vi "MAC6000_test.vi"() -> ()   [LabVIEW 2018, in "Stage Controller.lvlib"]
uses:
  <vilib>/Instr/_visa.llb/VISA Configure Serial Port (Instr).vi
  Stage Controller.lvlib
panel:
  out "COM Port":string
  in  "Status":bool
  in  "Controller Response":string
  in  "ABORT":bool
  in  "Tab Control":enum32{"Jump", "Home", "Scan"}(tab)
  in  "Step (um)":i32=100
  in  "Move Forward Button":bool
  in  "Move Back Button":bool
  in  "Next Lane Button":bool
  in  "Previous Lane Button":bool
  in  "Move Home":bool
  in  "Set Home":bool
  in  "Scan distance (um)":i32=1000
  in  "Scan Speed\n(pulses per sec)":u32=100 min=100 max=20000
  in  "Scan":bool
  in  "Exit":bool
  out "error out":errorcluster
  # "X Direction"
  # "µm"
  # "Y Direction"
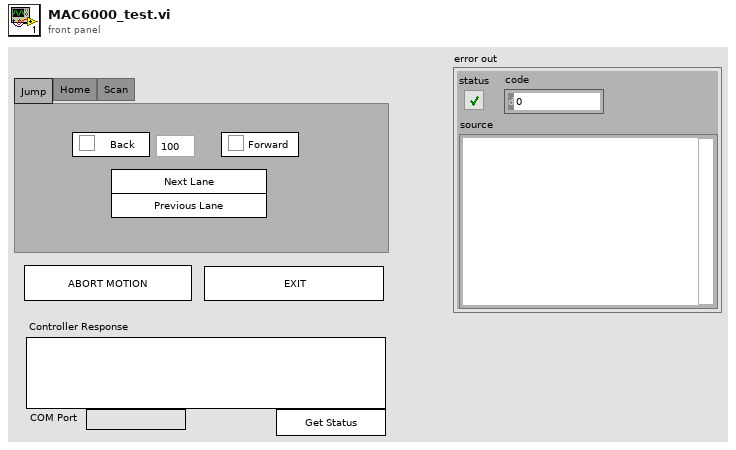
[diagram p1: front panel]
types:
  T1 = enum8{"Enabled", "Disabled", "Disabled and Grayed Out"}
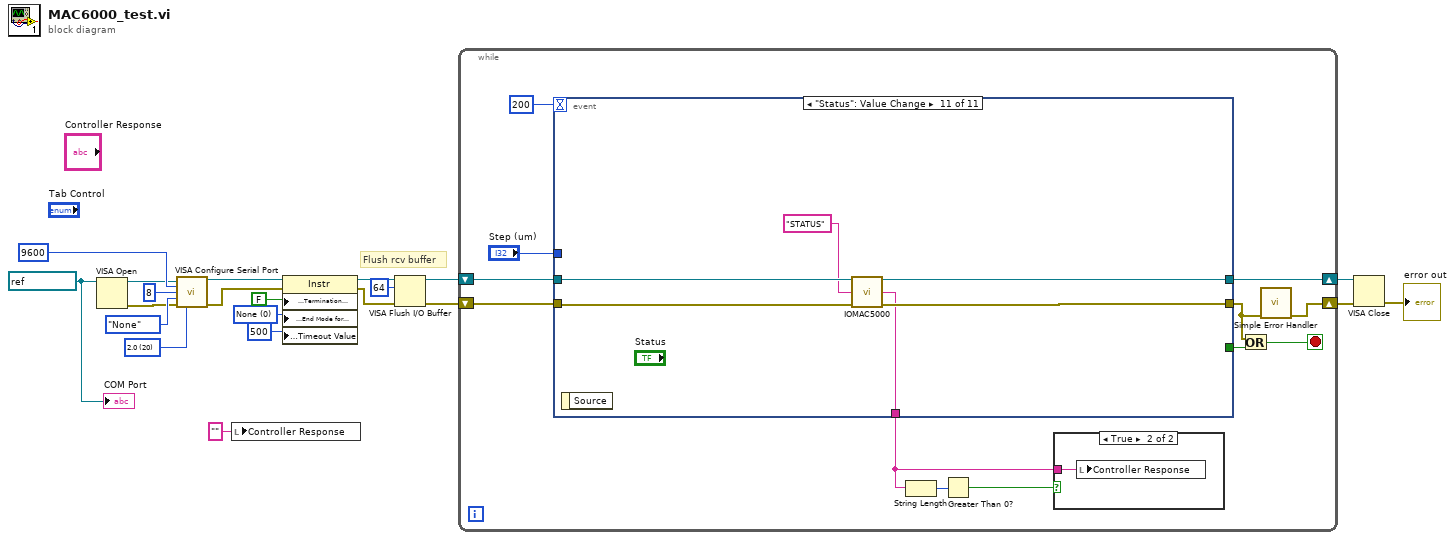
[diagram p0: block diagram]
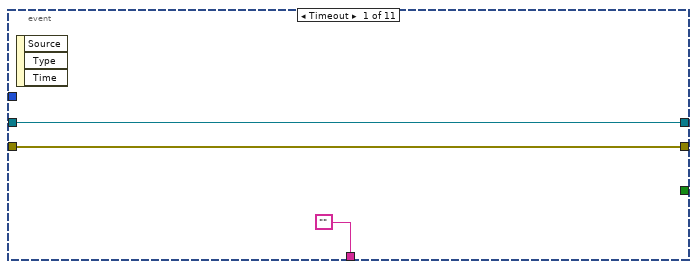
[diagram p3: hidden frame]
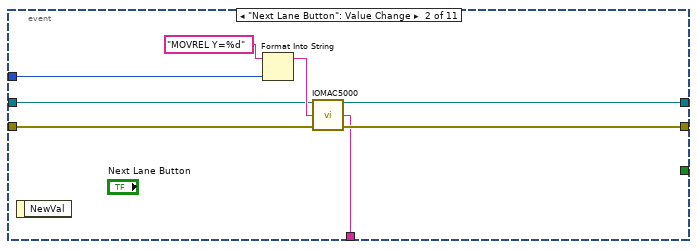
[diagram p4: hidden frame]
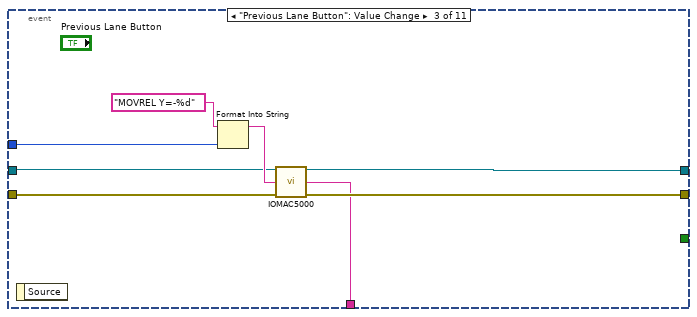
[diagram p5: hidden frame]
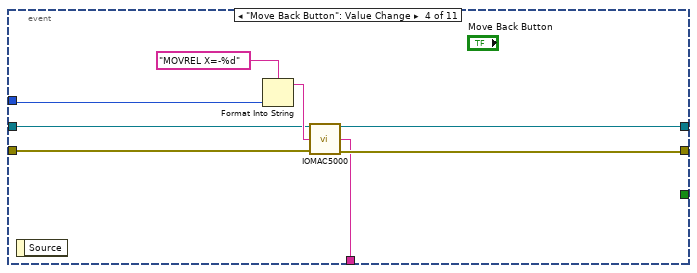
[diagram p6: hidden frame]
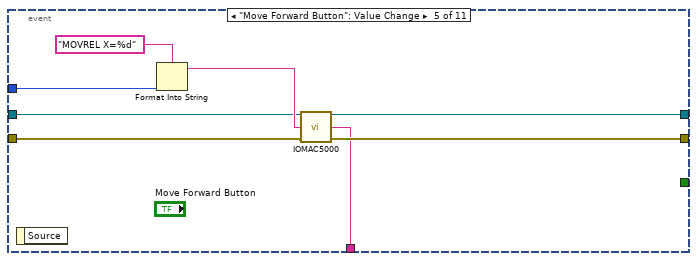
[diagram p7: hidden frame]
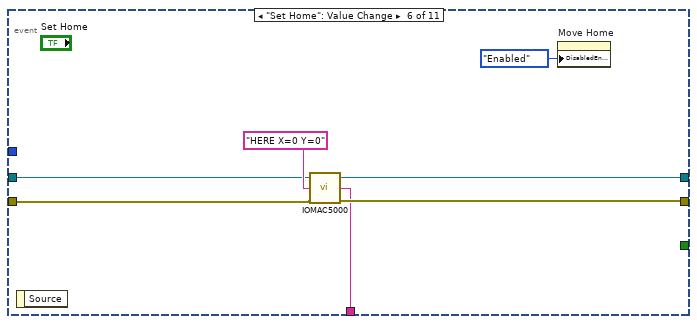
[diagram p8: hidden frame]
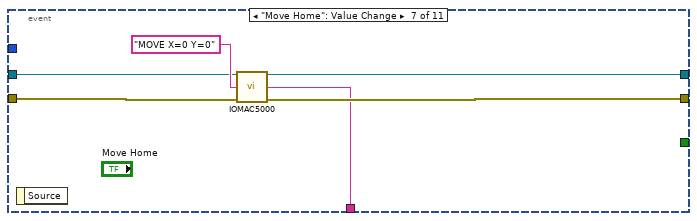
[diagram p9: hidden frame]
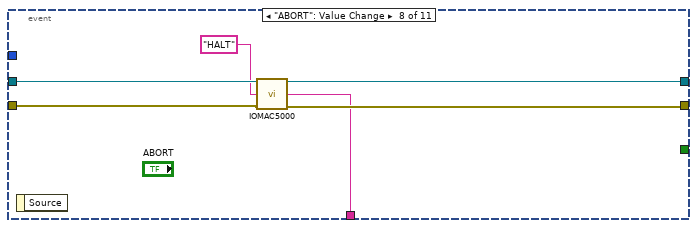
[diagram p10: hidden frame]
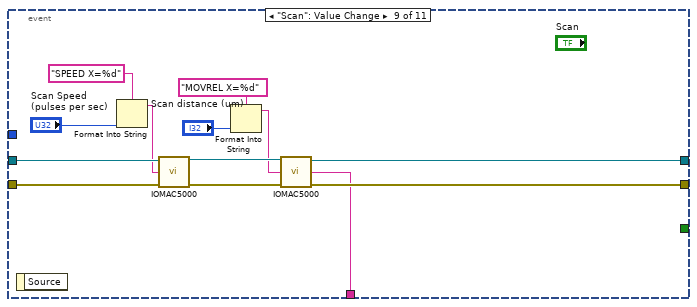
[diagram p11: hidden frame]
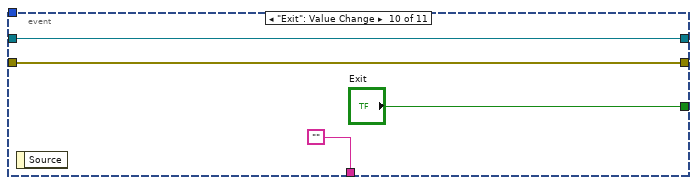
[diagram p12: hidden frame]
diagram:
  w1 = refnum<visa-resource-name> "COM10" ("COM Port")
  w8 = u16 20 items=["1.0"=10, "1.5"=15, "2.0"=20] ("stop bits (10: 1 bit)")
  w15 = u16 0 items=["None", "LastBit", "TermChar"] ("Serial Settings:Serial End Mode for Reads")
  # "Flush rcv buffer"
  n1 = VISA Open(VISA resource name=w1) -> (VISA resource name=w7:refnum<visa-resource-name>, error out=w6:errorcluster)  [unwired: 4 in]
  n2 = call-poly "VISA Configure Serial Port"("VISA resource name"=w7, "baud rate (9600)"=u32 9600 ("baud rate"), "data bits (8)"=u16 8, "parity (0:none)"=enum16{"None", "Odd", "Even", "Mark", "Space"}."None", "error in (no error)"=w6, "stop bits (10: 1 bit)"=w8) -> ("VISA resource name out"=w13:refnum<visa-resource-name>, "error out"=w12:errorcluster)  [unwired: 8 in]
  n3 = local write "Controller Response"("" ("Controller Response")) -> ()
  n4 = property class="Instr"(reference=w13, error in=w12, "Message Based Settings:Termination Character Enable"=FALSE, "Serial Settings:End Mode for Reads"=w15, "General Settings:Timeout Value"=u32 500) -> (reference out=w10:refnum<visa-resource-name>, error out=w9:errorcluster)
  n5 = VISA Flush I/O Buffer(VISA resource name=w10, mask (16)=u16 64, error in (no error)=w9) -> (VISA resource name out=w5:refnum<visa-resource-name>, error out=w4:errorcluster)
  n6 = while {
    shift-right: [w33] -> w20
    shift-left: w5 -> [w32]
    shift-right: [w25] -> w21
    shift-left: w4 -> [w31]
    stop <- w28 stop-if-true
    n7 = event shown="[10] \"Status\": Value Change" {
      selector: _ -> [_ _ _ _ _ _ _ _ _ _ _]
      dyn-events: _ -> [_ _ _ _ _ _ _ _ _ _ _]
      timeout: 200 -> [_ _ _ _ _ _ _ _ _ _ _]
      tunnel: [w36 w42 w48 w59 w66 w75 w82 w86 w93 w103 w109] -> w26
      tunnel: [w37 w43 w47 w58 w67 w74 w81 w85 w92 w104 w110] -> w33
      tunnel: w32 -> [w37 w40 w50 w56 w63 w72 w79 w88 w96 w104 w111]
      tunnel: w31 -> [w36 w39 w49 w55 w62 w71 w78 w87 w97 w103 w108]
      tunnel: "Step (um)" -> [_ w44 w52 w60 w68 _ _ _ _ _ _]
      tunnel: [_ _ _ _ _ _ _ _ _ "Exit" _] -> w29
      tunnel: ["" w38 w46 w54 w65 w70 w77 w83 w91 "" w106] -> w24
      event Timeout {
        n8 = event-data() -> ()  [unwired: 1 in, 3 out]
      }
      event "Next Lane Button": Value Change {
        n9 = event-data() -> ()  [unwired: 1 in, 1 out]
        n10 = Format Into String(format string="MOVREL Y=%d" ("string"), w44) -> (resulting string=w41:string)  [unwired: 2 in, 1 out]
        n11 = call "IOMAC5000.vi"("VISA  IN"=w40, "Command (to ctlr)"=w41, "error in"=w39) -> ("VISA OUT"=w43:refnum<visa-resource-name>, "Raw Response"=w38:string, "error out"=w42:errorcluster)  [unwired: 9 in, 1 out]
      }
      event "Previous Lane Button": Value Change {
        n12 = event-data() -> ()  [unwired: 1 in, 1 out]
        n13 = Format Into String(format string="MOVREL Y=-%d" ("string"), w52) -> (resulting string=w51:string)  [unwired: 2 in, 1 out]
        n14 = call "IOMAC5000.vi"("VISA  IN"=w50, "Command (to ctlr)"=w51, "error in"=w49) -> ("VISA OUT"=w47:refnum<visa-resource-name>, "Raw Response"=w46:string, "error out"=w48:errorcluster)  [unwired: 9 in, 1 out]
      }
      event "Move Back Button": Value Change {
        n15 = event-data() -> ()  [unwired: 1 in, 1 out]
        n16 = Format Into String(format string="MOVREL X=-%d" ("string"), w60) -> (resulting string=w57:string)  [unwired: 2 in, 1 out]
        n17 = call "IOMAC5000.vi"("VISA  IN"=w56, "Command (to ctlr)"=w57, "error in"=w55) -> ("VISA OUT"=w58:refnum<visa-resource-name>, "Raw Response"=w54:string, "error out"=w59:errorcluster)  [unwired: 9 in, 1 out]
      }
      event "Move Forward Button": Value Change {
        n18 = event-data() -> ()  [unwired: 1 in, 1 out]
        n19 = Format Into String(format string="MOVREL X=%d" ("string"), w68) -> (resulting string=w64:string)  [unwired: 2 in, 1 out]
        n20 = call "IOMAC5000.vi"("VISA  IN"=w63, "Command (to ctlr)"=w64, "error in"=w62) -> ("VISA OUT"=w67:refnum<visa-resource-name>, "Raw Response"=w65:string, "error out"=w66:errorcluster)  [unwired: 9 in, 1 out]
      }
      event "Set Home": Value Change {
        n21 = event-data() -> ()  [unwired: 1 in, 1 out]
        n22 = call "IOMAC5000.vi"("VISA  IN"=w72, "Command (to ctlr)"="HERE X=0 Y=0" ("true string"), "error in"=w71) -> ("VISA OUT"=w74:refnum<visa-resource-name>, "Raw Response"=w70:string, "error out"=w75:errorcluster)  [unwired: 9 in, 1 out]
        n23 = property on="Move Home" class="Bool"("DisabledEnum"=T1."Enabled" ("Disabled")) -> ()  [unwired: 2 in, 2 out]
      }
      event "Move Home": Value Change {
        n24 = event-data() -> ()  [unwired: 1 in, 1 out]
        n25 = call "IOMAC5000.vi"("VISA  IN"=w79, "Command (to ctlr)"="MOVE X=0 Y=0" ("true string"), "error in"=w78) -> ("VISA OUT"=w81:refnum<visa-resource-name>, "Raw Response"=w77:string, "error out"=w82:errorcluster)  [unwired: 9 in, 1 out]
      }
      event "ABORT": Value Change {
        n26 = event-data() -> ()  [unwired: 1 in, 1 out]
        n27 = call "IOMAC5000.vi"("VISA  IN"=w88, "Command (to ctlr)"="HALT" ("true string"), "error in"=w87) -> ("VISA OUT"=w85:refnum<visa-resource-name>, "Raw Response"=w83:string, "error out"=w86:errorcluster)  [unwired: 9 in, 1 out]
      }
      event "Scan": Value Change {
        n28 = event-data() -> ()  [unwired: 1 in, 1 out]
        n29 = Format Into String(format string="SPEED X=%d" ("string"), "Scan Speed\n(pulses per sec)") -> (resulting string=w90:string)  [unwired: 2 in, 1 out]
        n30 = call "IOMAC5000.vi"("VISA  IN"=w96, "Command (to ctlr)"=w90, "error in"=w97) -> ("VISA OUT"=w95:refnum<visa-resource-name>, "error out"=w94:errorcluster)  [unwired: 9 in, 2 out]
        n31 = Format Into String(format string="MOVREL X=%d" ("string"), "Scan distance (um)") -> (resulting string=w89:string)  [unwired: 2 in, 1 out]
        n32 = call "IOMAC5000.vi"("VISA  IN"=w95, "Command (to ctlr)"=w89, "error in"=w94) -> ("VISA OUT"=w92:refnum<visa-resource-name>, "Raw Response"=w91:string, "error out"=w93:errorcluster)  [unwired: 9 in, 1 out]
      }
      event "Exit": Value Change {
        n33 = event-data() -> ()  [unwired: 1 in, 1 out]
      }
      event "Status": Value Change {
        n34 = event-data() -> ()  [unwired: 1 in, 1 out]
        n35 = call "IOMAC5000.vi"("VISA  IN"=w111, "Command (to ctlr)"="STATUS", "error in"=w108) -> ("VISA OUT"=w110:refnum<visa-resource-name>, "Raw Response"=w106:string, "error out"=w109:errorcluster)  [unwired: 9 in, 1 out]
      }
    }
    n36 = String Length(string=w24) -> (length=w23:i32)
    n37 = Greater Than 0?(x=w23) -> (x > 0?=w22:bool)
    n38 = case shown="True" w22 {
      tunnel: w24 -> [_ w34]
      frame False {
      }
      frame True {
        n39 = local write "Controller Response"(w34) -> ()
      }
    }
    n40 = Or(x=w26, y=w29) -> (x .or. y?=w28:bool)
    n41 = call <vilib>:"Simple Error Handler.vi"("error in (no error)"=w26) -> ("error out"=w25:errorcluster)  [unwired: 4 in, 4 out]
  }
  n42 = VISA Close(VISA resource name=w20, error in (no error)=w21) -> (error out=→"error out":errorcluster)
  "COM Port" <- w1
